vi "Actor Core.vi"(8 "error in":errorcluster, 11 "Acquisition in":refnum<class "Acquisition.lvclass">) -> (0 "error out":errorcluster, 3 "Actor out":refnum<class "Actor.lvclass">)   [LabVIEW 2018, in "Acquisition.lvlib" / "Acquisition.lvclass"]
doc: "(<B>Filename</B>: Actor Framework.lvlib:Actor.lvclass:Actor Core.vi)\n\nReceives messages to the actor, reacts to them, and initiates any error handling that may shut the actor down.\n\nDescendant classes may override this VI to append parallel tasks for the actor to complete while it handles messages. Overrides use the Call Parent Method node."
uses:
  Acquisition.lvclass
  C:/Program Files (x86)/National Instruments/LabVIEW 2018/vi.lib/ActorFramework/Actor/Actor.lvclass
  <vilib>/ActorFramework/Actor/Actor.lvclass
  <vilib>/ActorFramework/Actor/Actor.lvclass/Actor.ctl
  Acquisition.lvclass/Acquisition.ctl
  Acquisition UI/Acquisition UI Messages/Display Data Msg/Display Data Msg.lvclass/Display Data Msg.ctl
  <vilib>/ActorFramework/Message Enqueuer/Message Enqueuer.lvclass/Message Enqueuer.ctl
  <vilib>/ActorFramework/Message Enqueuer/Enqueue.vi
  Acquisition UI/Acquisition UI Messages/Display Data Msg/Display Data Msg.lvclass
  C:/Program Files (x86)/National Instruments/LabVIEW 2018/vi.lib/ActorFramework/Message/Message.lvclass
  <vilib>/ActorFramework/Message Priority Queue/Priority Enqueue.vi
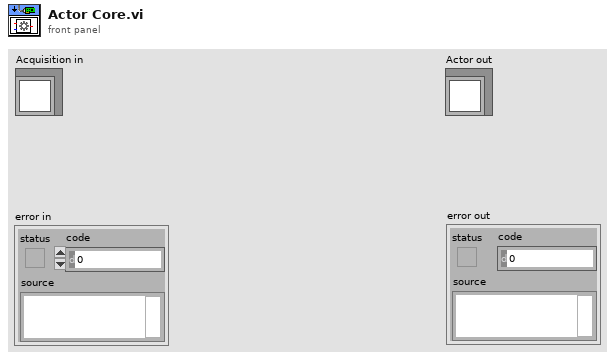
[diagram p1: front panel]
types:
  T1 = typedef "Acquisition.lvlib/Acquisition.lvclass/Helper Loop Events--cluster.ctl" = cluster{"Wake up":refnum<user-event>, "Put to Sleep":refnum<user-event>, "Exit":refnum<user-event>}
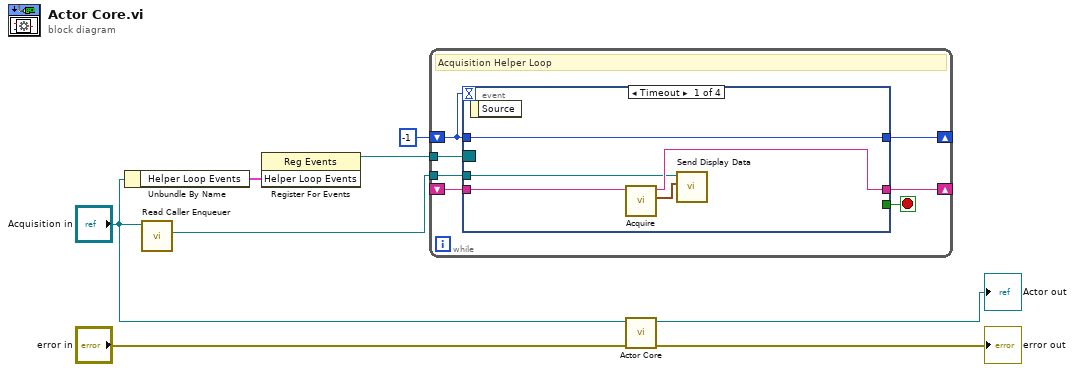
[diagram p0: block diagram]
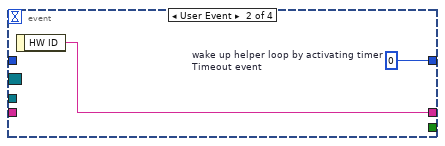
[diagram p2: hidden frame]
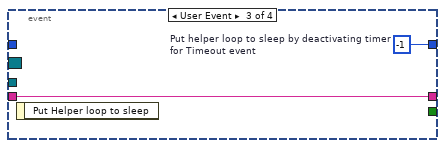
[diagram p3: hidden frame]
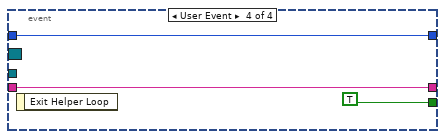
[diagram p4: hidden frame]
diagram:
  n1 = Unbundle By Name("Acquisition in") -> ("Helper Loop Events"=w5:T1)
  n2 = call <vilib>:"Read Caller Enqueuer.vi"("Actor"="Acquisition in") -> ("Caller Enqueuer"=w1:refnum<class "Message Enqueuer.lvclass">)  [unwired: 10 in]
  n3 = register-events(w5) -> (reference out=w4:refnum<event-registration>)  [unwired: 2 in, 1 out]
  n4 = while {
    tunnel: w4 -> [w15]
    shift-right: [w13] -> _
    shift-left: -1 -> [w12]
    shift-right: [w11] -> _
    shift-left: _ -> [w10]
    tunnel: w1 -> [w9]
    stop <- w14 stop-if-true
    # "Acquisition Helper Loop"
    n5 = event shown="[0] Timeout" {
      selector: w15 -> [_ _ _ _]
      dyn-events: _ -> [_ _ _ _]
      timeout: w12 -> [_ _ _ _]
      tunnel: [_ _ _ TRUE] -> w14
      tunnel: [w20 w22 w24 w26] -> w13
      tunnel: w12 -> [w20 _ _ w26]
      tunnel: [w18 w21 w23 w25] -> w11
      tunnel: w10 -> [w19 _ w23 w25]
      tunnel: w9 -> [w16 _ _ _]
      event Timeout {
        n6 = event-data() -> ()  [unwired: 1 in, 1 out]
        n7 = call "Acquire.vi"("HW ID in"=w19) -> ("Graph Data"=w17:waveform(dbl)[], "HW ID out"=w18:string)  [unwired: 8 in, 1 out]
        n8 = call "Send Display Data.vi"("Graph Data"=w17, "Message Enqueuer"=w16) -> ()  [unwired: 8 in, 2 out]
      }
      event User Event {
        w22 = 0  # wake up helper loop by activating timer Timeout event
        n9 = event-data() -> ("HW ID"=w21:string)  [unwired: 1 in]
      }
      event User Event {
        w24 = -1  # Put helper loop to sleep by deactivating timer for Timeout event
        n10 = event-data() -> ()  [unwired: 1 in, 1 out]
      }
      event User Event {
        n11 = event-data() -> ()  [unwired: 1 in, 1 out]
      }
    }
  }
  n12 = call-parent "Actor Core.vi"("error in"="error in", "Actor in"="Acquisition in") -> ("error out"=→"error out":errorcluster, "Actor out"=→"Actor out":refnum<class "Actor.lvclass">)  [unwired: 8 in]
